vi "lvpeak_list_cameras.vi"(8 "error in (no error)":errorcluster) -> (0 "error out":errorcluster, 3 "LVPeak Cameras":T1[](array[typedef]))   [LabVIEW 2024, in "Vision.lvlib"]
uses:
  Vision.lvlib
  lvpeak_camera.ctl
  bin/LVPeak.dll
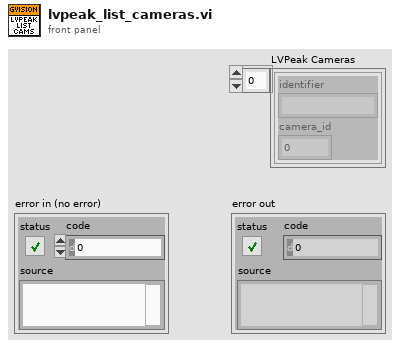
[diagram p1: front panel]
types:
  T1 = typedef "Vision.lvlib/lvpeak_camera.ctl" = cluster{"identifier":string, "camera_id":u64}
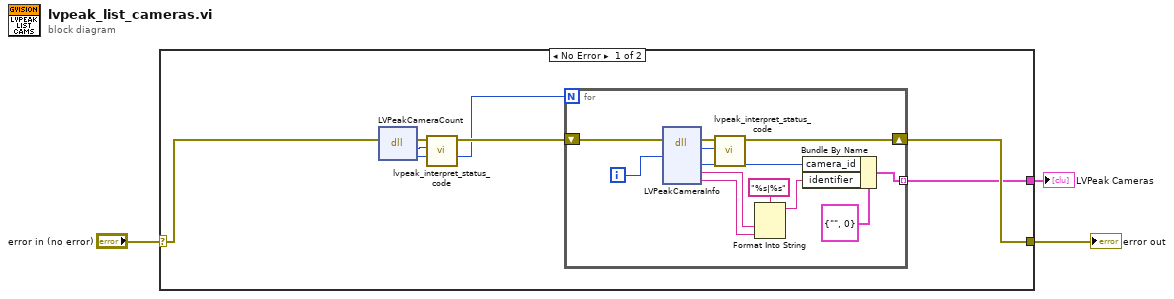
[diagram p0: block diagram]
diagram:
  n1 = case shown="No Error" "error in (no error)" {
    selector: "error in (no error)" -> [w10 w23]
    tunnel: [w5 w23] -> w2
    tunnel: [w4 _] -> w1
    frame No Error {
      n2 = dll-call lib="C:/Users/cfang/Desktop/nebraska-silicon-lab/pixel-gantry-control/Gantry/Shared Components/bin/LVPeak.dll" fn="LVPeakCameraCount"(error in=w10) -> (error out=w9:errorcluster, "return type"=w8:i32, "count"=w6:i32)  [unwired: 3 in, 1 out]
      n3 = call "lvpeak_interpret_status_code.vi"("status_code"=w8, "error in (no error)"=w9) -> ("error out"=w7:errorcluster)  [unwired: 9 in]
      n4 = for {
        N: w6 -> [_]
        shift-right: [w19] -> w5
        shift-left: w7 -> [w22]
        tunnel: [w16] -> w4 mode=indexing
        i -> [w18]
        n5 = dll-call lib="C:/Users/cfang/Desktop/nebraska-silicon-lab/pixel-gantry-control/Gantry/Shared Components/bin/LVPeak.dll" fn="LVPeakCameraInfo"(error in=w22, "cam_idx"=w18) -> (error out=w21:errorcluster, "return type"=w20:i32, "camera_id"=w15:u64, "cam_name"=w13:string, "serial_number"=w12:string)  [unwired: 6 in, 1 out]
        n6 = call "lvpeak_interpret_status_code.vi"("status_code"=w20, "error in (no error)"=w21) -> ("error out"=w19:errorcluster)  [unwired: 9 in]
        n7 = Format Into String(format string="%s|%s", w13, w12) -> (resulting string=w11:string)  [unwired: 2 in, 1 out]
        n8 = Bundle By Name(cluster=T1 {"identifier"="", "camera_id"=0}, "camera_id"=w15, "identifier"=w11) -> (w16:T1)
      }
    }
    frame Error {
    }
  }
  "error out" <- w2
  "LVPeak Cameras" <- w1
